vi "Water Fall A.vi"(11 "GIC Input":T1={"     Use ?\nOff       On"=[FALSE, TRUE, FALSE, TRUE], "Mode:"=FALSE, "Extra Port"="", "Hokuyo Port"="COM7", "Tx Prop  Port"="COM6", "Compass Port"="", "GPS Port"="", "Num of WPs"=0, "WP Lats and Longs"={"WP Lats"=[], "WP Longs"=[]}, "Obst Lats and Longs"={"Obst Lats"=[], "Obst Longs"=[]}, "Parameters"=[], "GPS Data"=[], "Compass"=0.0, "LMS Vector"=[], "Vision Vector"=[], "Direction Cmd"=0.0, "Speed Cmd"=0.0, "WP Vector"=[], "WP Number"=0, "Extra"=0, "SW Map"=[], "Path Cluster"={"Path x node"=[], "Path y node"=[]}, "Sim Course"=[]} {"Obst Lats and Longs"."Obst Longs" format="%#_8g"; "Obst Lats and Longs"."Obst Lats" format="%#_8g"}) -> (3 "GIC Output":T1={"     Use ?\nOff       On"=[FALSE, TRUE, FALSE, TRUE], "Mode:"=FALSE, "Extra Port"="", "Hokuyo Port"="COM7", "Tx Prop  Port"="COM6", "Compass Port"="", "GPS Port"="", "Num of WPs"=0, "WP Lats and Longs"={"WP Lats"=[], "WP Longs"=[]}, "Obst Lats and Longs"={"Obst Lats"=[], "Obst Longs"=[]}, "Parameters"=[], "GPS Data"=[], "Compass"=0.0, "LMS Vector"=[], "Vision Vector"=[], "Direction Cmd"=0.0, "Speed Cmd"=0.0, "WP Vector"=[], "WP Number"=0, "Extra"=0, "SW Map"=[], "Path Cluster"={"Path x node"=[], "Path y node"=[]}, "Sim Course"=[]} {"Obst Lats and Longs"."Obst Longs" format="%#_8g"; "Obst Lats and Longs"."Obst Lats" format="%#_8g"})   [LabVIEW 2014]
panel:
  out "test3":dbl
  out "Test2":dbl
  in  "Test Parameters":dbl[](array[numeric])
  out "Numeric":dbl
  # "Water Fall A"
  # "Input:"
  # "Output"
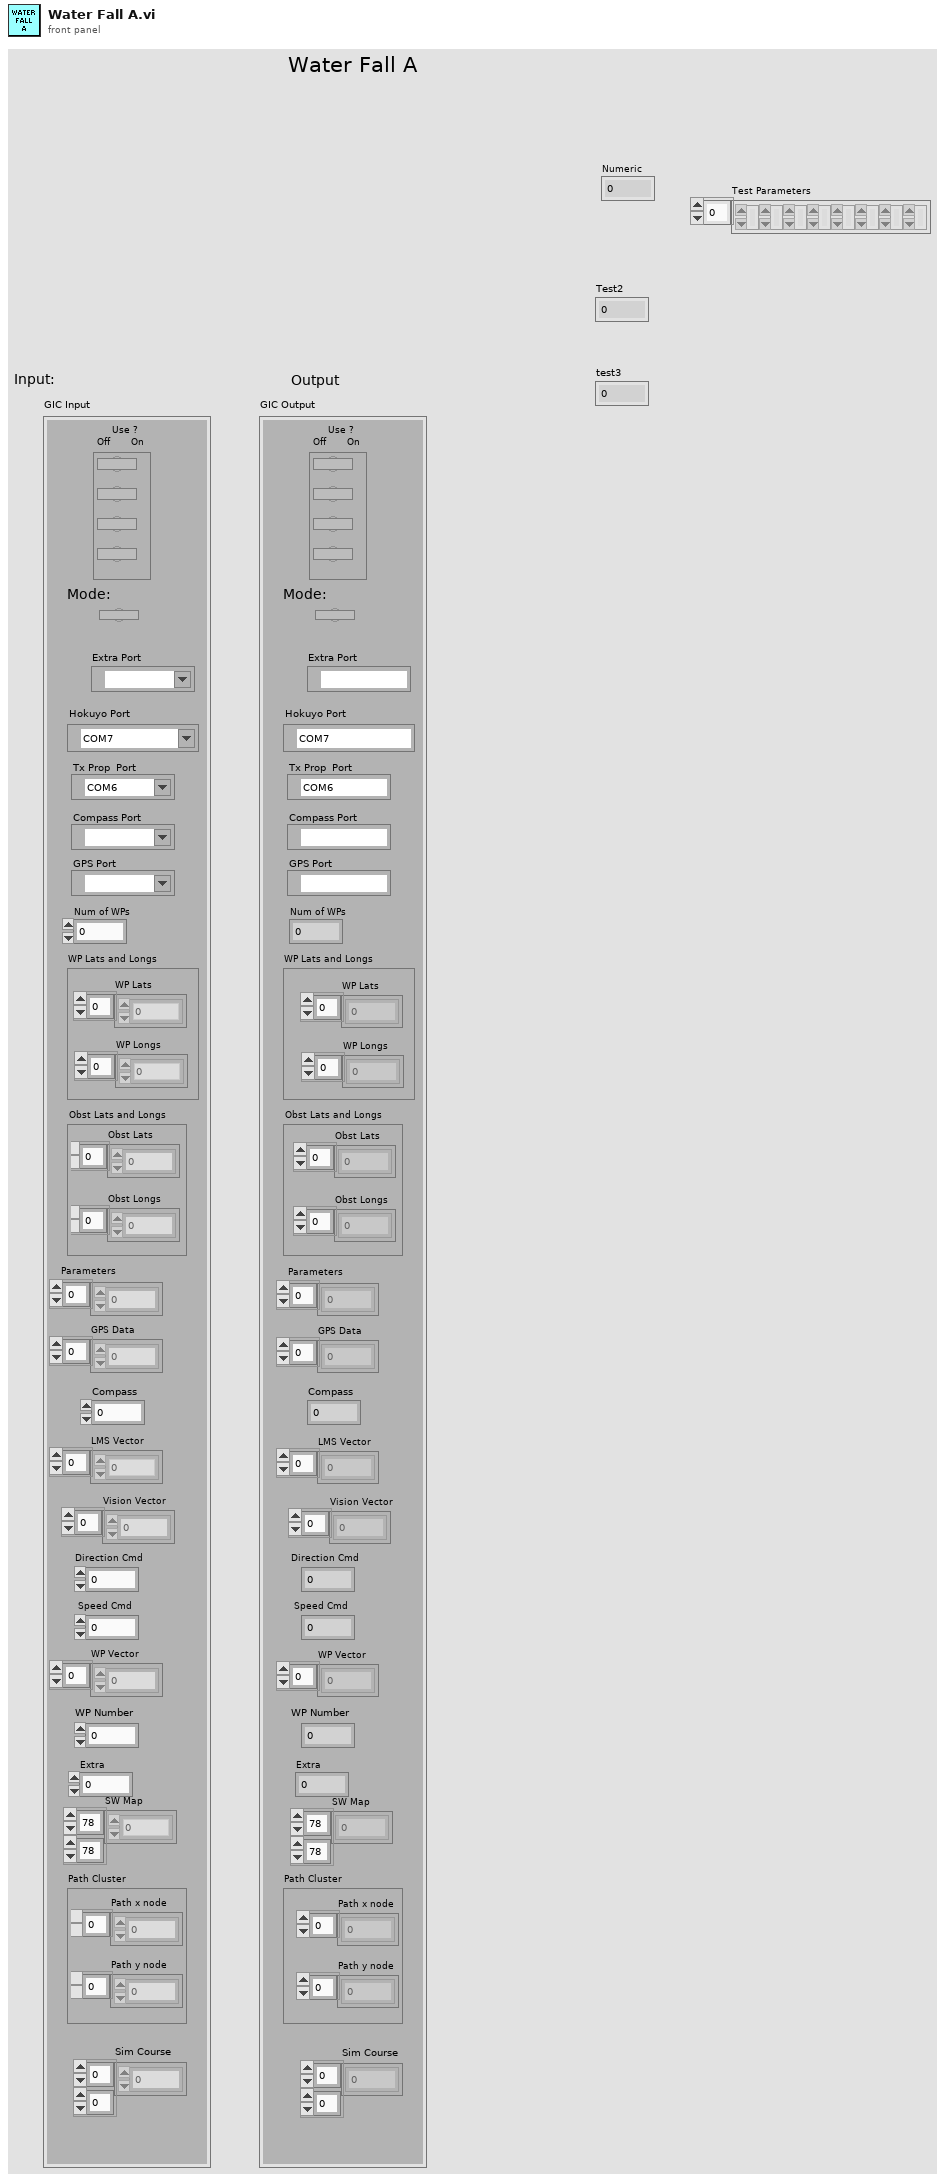
[diagram p1: front panel]
types:
  T1 = cluster{"     Use ?\nOff       On":bool[], "Mode:":bool, "Extra Port":refnum<visa-resource-name>, "Hokuyo Port":refnum<visa-resource-name>, "Tx Prop  Port":refnum<visa-resource-name>, "Compass Port":refnum<visa-resource-name>, "GPS Port":refnum<visa-resource-name>, "Num of WPs":i16, "WP Lats and Longs":cluster{"WP Lats":dbl[], "WP Longs":dbl[]}, "Obst Lats and Longs":cluster{"Obst Lats":dbl[], "Obst Longs":dbl[]}, "Parameters":dbl[], "GPS Data":dbl[], "Compass":dbl, "LMS Vector":dbl[], "Vision Vector":dbl[], "Direction Cmd":dbl, "Speed Cmd":dbl, "WP Vector":dbl[], "WP Number":i32, "Extra":i16, "SW Map":i32[][], "Path Cluster":cluster{"Path x node":dbl[], "Path y node":dbl[]}, "Sim Course":i8[][]}
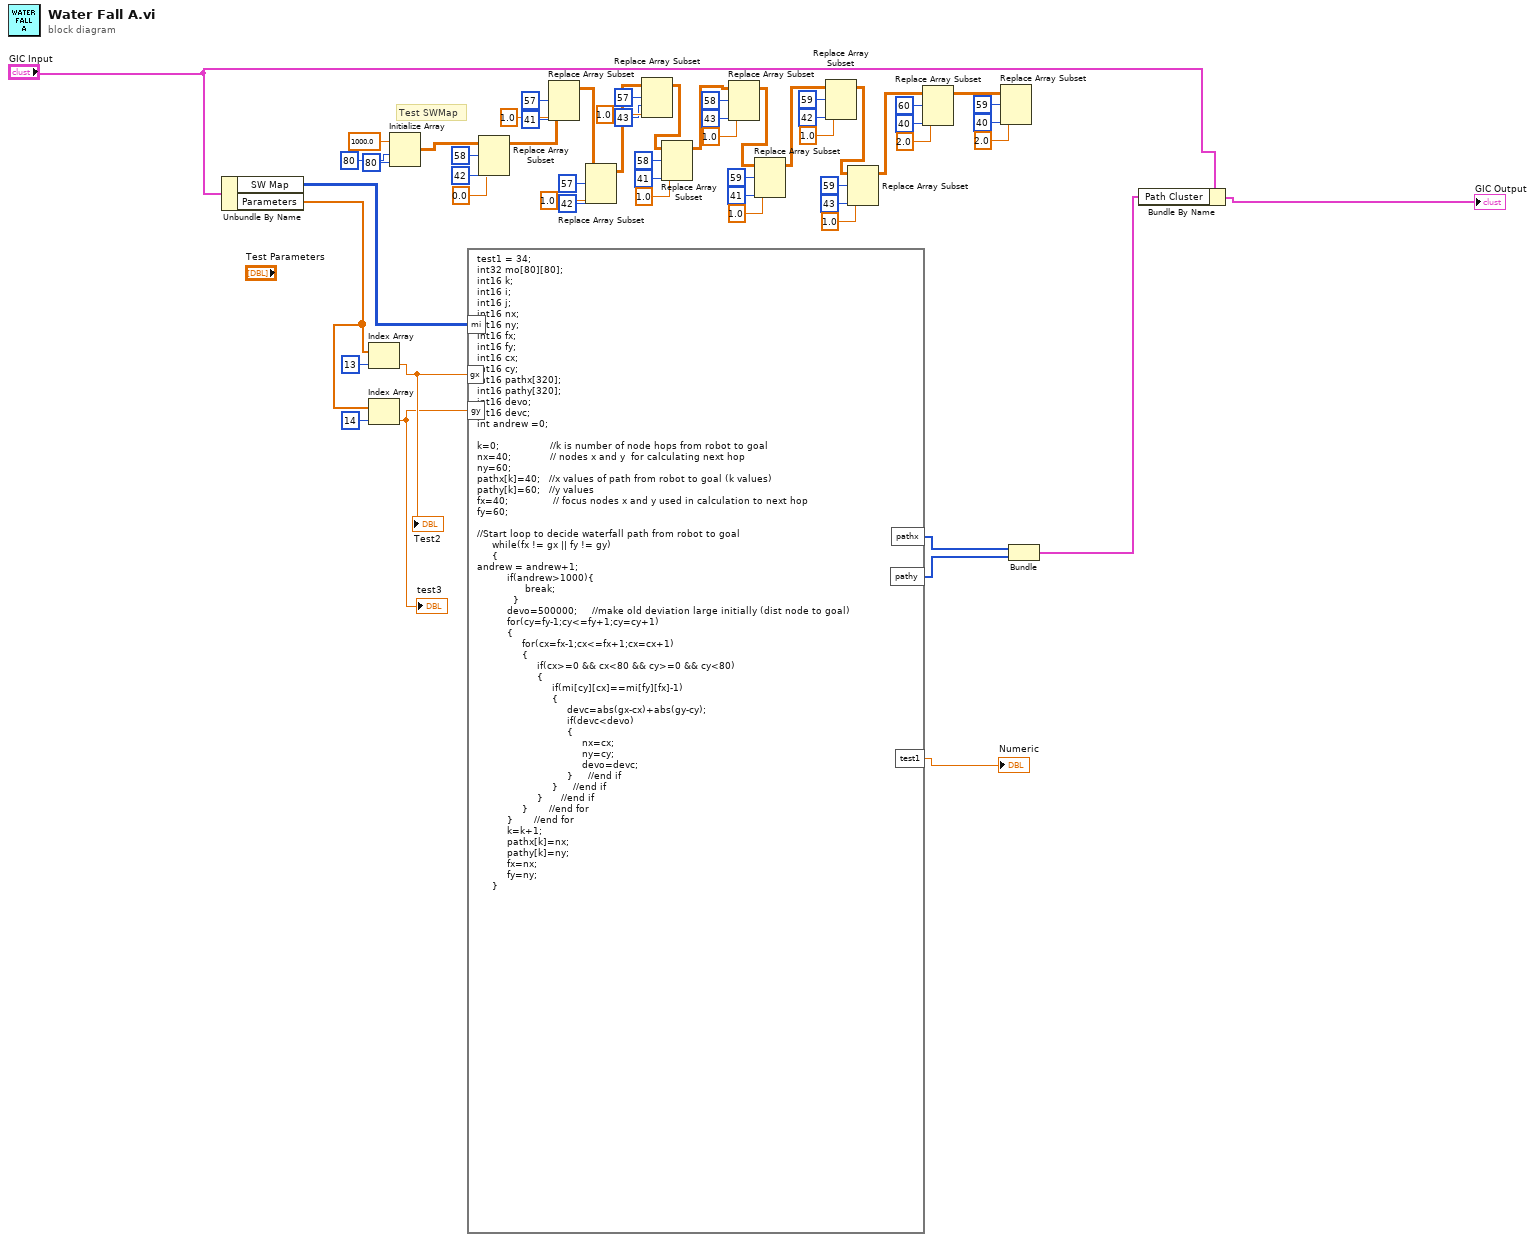
[diagram p0: block diagram]
diagram:
  # "Test SWMap"
  n1 = Unbundle By Name("GIC Input") -> ("SW Map"=w41:i32[][], "Parameters"=w42:dbl[])
  n2 = Index Array(array=w42, index=13) -> (element=w7:dbl)
  "Test2" <- w7
  n3 = Index Array(array=w42, index=14) -> (element=w6:dbl)
  "test3" <- w6
  n4 = Initialize Array(1000.0 ("element"), 80 ("dimension size"), 80 ("dimension size")) -> (w56:dbl[][])
  n5 = formula code="test1 = 34;\nint32 mo[80][80];\nint16 k;\nint16 i;\nint16 j;\nint16 nx;\nint16 ny;\nint16 fx;\nint16 fy;\nint16 cx;\nint16 cy;\nint16 pathx[320];\nint16 pathy[320];\nint16 devo;\nint16 devc;\nint andrew =0;\n\nk=0;                 //k is number of node hops from robot to goal\nnx=40;             // nodes x and y  for calculating next hop\nny=60;\npathx[k]=40;   //x values of path from robot to goal (k values)\npathy[k]=60;   //y values\nfx=40;               // focus nodes x and y used in calculation to next hop\nfy=60;\n\n//Start loop to decide waterfall path from robot to goal\n     while(fx != gx || fy != gy)\n     {\nandrew = andrew+1;\n          if(andrew>1000){\n                break;\n            }\n          devo=500000;     //make old deviation large initially (dist node to goal)\n          for(cy=fy-1;cy<=fy+1;cy=cy+1)\n          {\n               for(cx=fx-1;cx<=fx+1;cx=cx+1)\n               {\n                    if(cx>=0 && cx<80 && cy>=0 && cy<80)\n                    {\n                         if(mi[cy][cx]==mi[fy][fx]-1)\n                         {\n                              devc=abs(gx-cx)+abs(gy-cy);\n                              if(devc<devo)\n                              {\n                                   nx=cx;\n                                   ny=cy;\n                                   devo=devc;\n                              }     //end if\n                         }     //end if\n                    }      //end if\n               }       //end for\n          }       //end for\n          k=k+1;\n          pathx[k]=nx;\n          pathy[k]=ny;\n          fx=nx;\n          fy=ny;\n     }"("mi"=w41, "gx"=w7, "gy"=w6) -> ("test1"=→"Numeric":dbl, "pathx"=w5:i16[], "pathy"=w4:i16[])
  n6 = Replace Array Subset(array=w56, new element=0.0 ("new element/subarray"), index (row)=58, index (col)=42 ("disabled index (col)")) -> (w52:dbl[][])
  n7 = Replace Array Subset(array=w52, new element=1.0 ("new element/subarray"), index (row)=57, index (col)=41 ("disabled index (col)")) -> (w48:dbl[][])
  n8 = Replace Array Subset(array=w48, new element=1.0 ("new element/subarray"), index (row)=57, index (col)=42 ("disabled index (col)")) -> (w40:dbl[][])
  n9 = Replace Array Subset(array=w40, new element=1.0 ("new element/subarray"), index (row)=57, index (col)=43 ("disabled index (col)")) -> (w36:dbl[][])
  n10 = Replace Array Subset(array=w36, new element=1.0 ("new element/subarray"), index (row)=58, index (col)=41 ("disabled index (col)")) -> (w32:dbl[][])
  n11 = Replace Array Subset(array=w32, new element=1.0 ("new element/subarray"), index (row)=58, index (col)=43 ("disabled index (col)")) -> (w28:dbl[][])
  n12 = Replace Array Subset(array=w28, new element=1.0 ("new element/subarray"), index (row)=59, index (col)=41 ("disabled index (col)")) -> (w24:dbl[][])
  n13 = Replace Array Subset(array=w24, new element=1.0 ("new element/subarray"), index (row)=59, index (col)=42 ("disabled index (col)")) -> (w20:dbl[][])
  n14 = Replace Array Subset(array=w20, new element=1.0 ("new element/subarray"), index (row)=59, index (col)=43 ("disabled index (col)")) -> (w16:dbl[][])
  n15 = Replace Array Subset(array=w16, new element=2.0 ("new element/subarray"), index (row)=60, index (col)=40 ("disabled index (col)")) -> (w12:dbl[][])
  n16 = Replace Array Subset(array=w12, new element=2.0 ("new element/subarray"), index (row)=59, index (col)=40 ("disabled index (col)")) -> ()  [unwired: 1 out]
  n17 = Bundle(w5, w4) -> (w3:cluster{i16[], i16[]})  [unwired: 1 in]
  n18 = Bundle By Name(cluster="GIC Input", "Path Cluster"=w3) -> (→"GIC Output":T1)
